vi "okCFrontPanelDevices Get Device Info.vi"(8 "error in (no error)":errorcluster, 11 "okCFrontPanel Device Refnum":refnum<k24>) -> (0 "error out":errorcluster, 2 "Device Info":T1, 3 "okCFrontPanel Device Refnum":refnum<k24>)   [LabVIEW 2021, in "okFrontPanelC#Wrapper.lvlib"]
uses:
  okFrontPanelC#Wrapper.lvlib
  D:/UCLA Thinkpad Google Drive/LabVIEW 2021 SP1/builds/SwissSPAD Live Distribution/Opal Kelly/C# Wrapper/v5.0.2/libFrontPanel-csharp.dll
  v5.0.2/libFrontPanel-csharp.dll
  okTDeviceInfo Struct.ctl
  okEDeviceInterface.ctl
  okTFlashLayoutStruct.ctl
  okTProductID.ctl
  okEUSBSpeed.ctl
panel:
  out "GetDeviceInfo":i32(ring) items=["NoError"=0, "InvalidParameter"=-20, "InvalidResetProfile"=-19, "DataAlignmentError"=-18, "FIFOOverflow"=-17, "FIFOUnderflow"=-16, "UnsupportedFeature"=-15, "I2CUnknownStatus"=-14, "I2CNack"=-13, "I2CBitError"=-12, "I2CRestrictedAddress"=-11, "InvalidBlockSize"=-10, "InvalidEndpoint"=-9, "DeviceNotOpen"=-8, "FileError"=-7, "InvalidBitstream"=-6, "CommunicationError"=-5, "TransferError"=-4, "DoneNotHigh"=-3, "Timeout"=-2, "Failed"=-1]
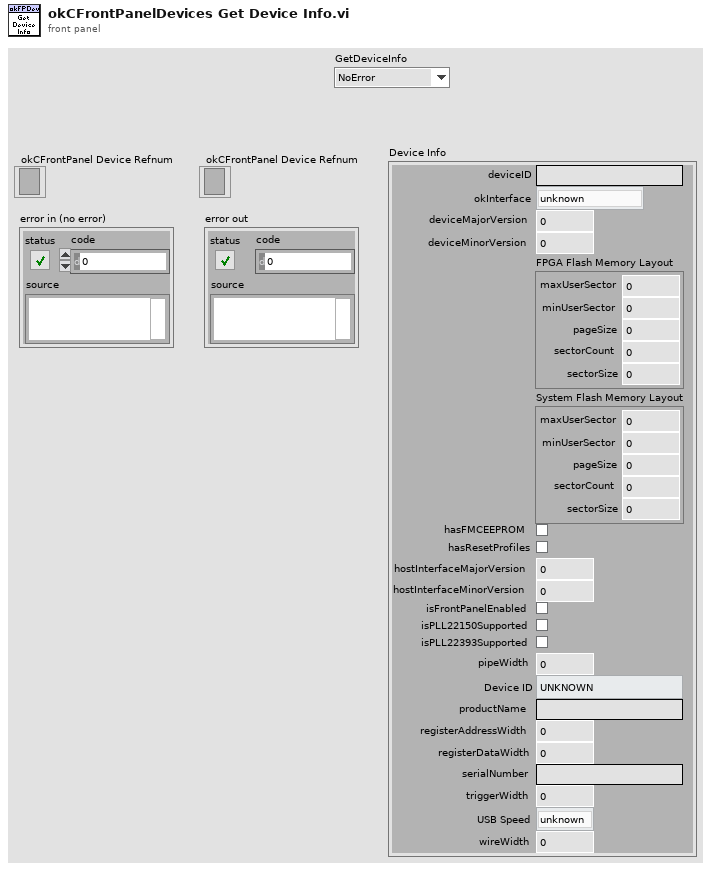
[diagram p1: front panel]
types:
  T1 = typedef "okFrontPanelC#Wrapper.lvlib/okTDeviceInfo Struct.ctl" = cluster{"deviceID":string, "okInterface":T2, "deviceMajorVersion":i32, "deviceMinorVersion":i32, "FPGA Flash Memory Layout":T3, "System Flash Memory Layout":T3, "hasFMCEEPROM":bool, "hasResetProfiles":bool, "hostInterfaceMajorVersion":i32, "hostInterfaceMinorVersion":i32, "isFrontPanelEnabled":bool, "isPLL22150Supported":bool, "isPLL22393Supported":bool, "pipeWidth":i32, "Device ID":T4, "productName":string, "registerAddressWidth":i32, "registerDataWidth":i32, "serialNumber":string, "triggerWidth":i32, "USB Speed":T5, "wireWidth":i32}
  T2 = typedef "okFrontPanelC#Wrapper.lvlib/okEDeviceInterface.ctl" = enum16{"unknown", "USB2", "PCIe", "USB3"}
  T3 = typedef "okFrontPanelC#Wrapper.lvlib/okTFlashLayoutStruct.ctl" = cluster{"maxUserSector":u32, "minUserSector":u32, "pageSize":u32, "sectorCount":u32, "sectorSize":u32}
  T4 = typedef "okFrontPanelC#Wrapper.lvlib/okTProductID.ctl" = enum16{"UNKNOWN", "XEM3001V1", "XEM3001V2", "XEM3010", "XEM3005", "XEM3001CL", "XEM3020", "XEM3050", "XEM9002", "XEM3001RB", "XEM5010", "XEM6110LX45", "XEM6001", "XEM6010LX45", "XEM6010LX150", "XEM6110LX150", "XEM6006LX9", "XEM6006LX16", "XEM6006LX25", "XEM5010LX110", "ZEM4310", "XEM6310LX45", "XEM6310LX150", "XEM6110V2LX45", "XEM6110V2LX150", "XEM6002LX9", "XEM6310MTLX45T", "XEM6320LX130T", "XEM7350K70T", "XEM7350K160T", "XEM7350K410T", "XEM6310MTLX150T", "ZEM5305A2", "ZEM5305A7", "XEM7001A15", "XEM7001A35", "XEM7360K160T", "XEM7360K410T", "ZEM5310A4", "ZEM5310A7", "ZEM5370A5", "XEM7010A50", "XEM7010A200", "XEM7310A75", "XEM7310A200", "XEM7320A75T", "XEM7320A200T", "XEM7305", "FPXBARE"}
  T5 = typedef "okFrontPanelC#Wrapper.lvlib/okEUSBSpeed.ctl" = enum16{"unknown", "Full", "High", "Super"}
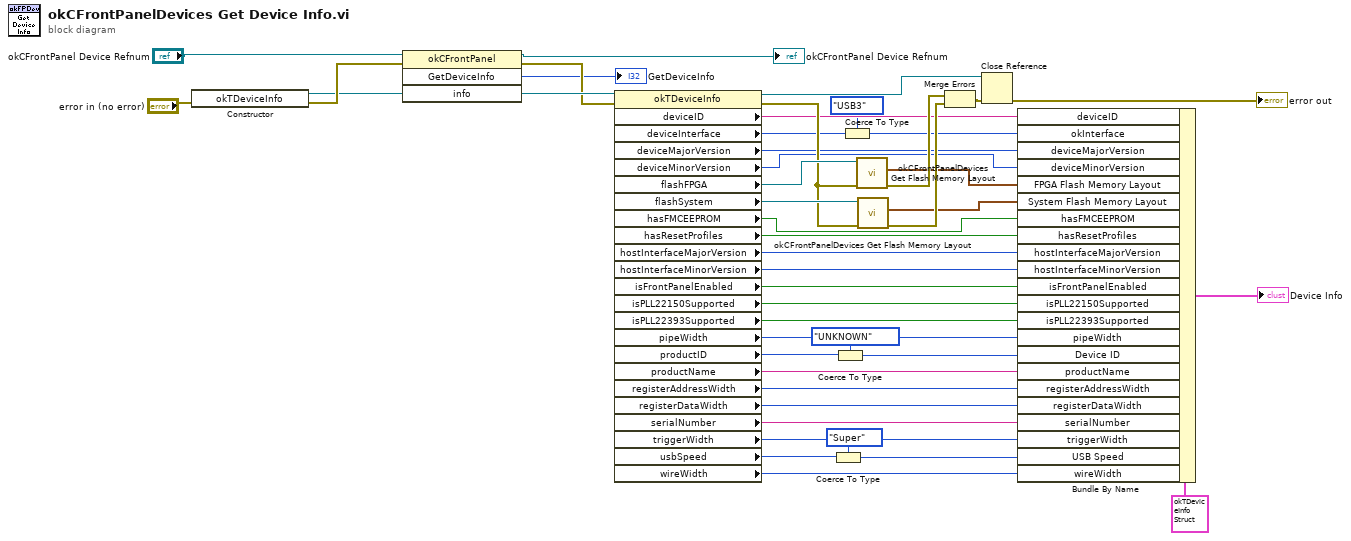
[diagram p0: block diagram]
diagram:
  n1 = constructor class="okTDeviceInfo"(error in="error in (no error)") -> (reference out=w41:refnum<k24>, error out=w42:errorcluster)  [unwired: 2 in, 1 out]
  n2 = invoke class="okCFrontPanel" method="GetDeviceInfo"(reference="okCFrontPanel Device Refnum", error in=w42, "info"=w41) -> (reference out=→"okCFrontPanel Device Refnum":refnum<k24>, error out=w40:errorcluster, "GetDeviceInfo"=→"GetDeviceInfo":i32)  [unwired: 1 in, 1 out]
  n3 = property class="okTDeviceInfo"(reference=w41, error in=w40) -> (reference out=w39:refnum<k24>, error out=w34:errorcluster, "deviceID"=w31:string, "deviceInterface"=w30:i32, "deviceMajorVersion"=w23:i32, "deviceMinorVersion"=w22:i32, "flashFPGA"=w37:refnum<k24>, "flashSystem"=w36:refnum<k24>, "hasFMCEEPROM"=w18:bool, "hasResetProfiles"=w19:bool, "hostInterfaceMajorVersion"=w17:i32, "hostInterfaceMinorVersion"=w16:i32, "isFrontPanelEnabled"=w15:bool, "isPLL22150Supported"=w14:bool, "isPLL22393Supported"=w13:bool, "pipeWidth"=w12:i32, "productID"=w25:i32, "productName"=w10:string, "registerAddressWidth"=w9:i32, "registerDataWidth"=w8:i32, "serialNumber"=w7:string, "triggerWidth"=w6:i32, "usbSpeed"=w27:i32, "wireWidth"=w4:i32)
  n4 = Coerce To Type(0:w27, 1:okEUSBSpeed."Super") -> (2:w5:T5)
  n5 = Coerce To Type(0:w25, 1:okTProductID."UNKNOWN") -> (2:w11:T4)
  n6 = Coerce To Type(0:w30, 1:okEDeviceInterface."USB3" ("okInterface")) -> (2:w29:T2)
  n7 = call "okCFrontPanelDevices Get Flash Memory Layout.vi"("error in (no error)"=w34, "okTFlashLayout Refnum"=w37) -> ("error out"=w35:errorcluster, "Flash Memory Layout"=w21:T3)  [unwired: 8 in]
  n8 = call "okCFrontPanelDevices Get Flash Memory Layout.vi"("error in (no error)"=w34, "okTFlashLayout Refnum"=w36) -> ("error out"=w33:errorcluster, "Flash Memory Layout"=w20:T3)  [unwired: 8 in]
  n9 = Merge Errors(w35, w33) -> (w32:errorcluster)
  n10 = Close Reference(reference=w39, error in (no error)=w32) -> (error out=→"error out":errorcluster)
  n11 = Bundle By Name(cluster=T1 {"deviceID"="", "okInterface"=enum."unknown", "deviceMajorVersion"=0, "deviceMinorVersion"=0, "FPGA Flash Memory Layout"={"maxUserSector"=0, "minUserSector"=0, "pageSize"=0, "sectorCount"=0, "sectorSize"=0}, "System Flash Memory Layout"={"maxUserSector"=0, "minUserSector"=0, "pageSize"=0, "sectorCount"=0, "sectorSize"=0}, "hasFMCEEPROM"=FALSE, "hasResetProfiles"=FALSE, "hostInterfaceMajorVersion"=0, "hostInterfaceMinorVersion"=0, "isFrontPanelEnabled"=FALSE, "isPLL22150Supported"=FALSE, "isPLL22393Supported"=FALSE, "pipeWidth"=0, "Device ID"=enum."UNKNOWN", "productName"="", "registerAddressWidth"=0, "registerDataWidth"=0, "serialNumber"="", "triggerWidth"=0, "USB Speed"=enum."unknown", "wireWidth"=0} ("Device Info"), "deviceID"=w31, "okInterface"=w29, "deviceMajorVersion"=w23, "deviceMinorVersion"=w22, "FPGA Flash Memory Layout"=w21, "System Flash Memory Layout"=w20, "hasFMCEEPROM"=w18, "hasResetProfiles"=w19, "hostInterfaceMajorVersion"=w17, "hostInterfaceMinorVersion"=w16, "isFrontPanelEnabled"=w15, "isPLL22150Supported"=w14, "isPLL22393Supported"=w13, "pipeWidth"=w12, "Device ID"=w11, "productName"=w10, "registerAddressWidth"=w9, "registerDataWidth"=w8, "serialNumber"=w7, "triggerWidth"=w6, "USB Speed"=w5, "wireWidth"=w4) -> (→"Device Info":T1)
